vi "VI Server - 호출대상.vi"(7 "dB On (F)":bool caption="dB On (거짓)", 9 "export mode":T1 caption="반출 모드" items=["파워 스펙트럼", "파워 스펙트럼 밀도"], 10 "window":T2=1 caption="윈도우" items=["사각형"=0, "해닝"=1, "해밍"=2, "블랙맨-해리스"=3, "정밀한 블랙맨"=4, "블랙맨"=5, "플랫 탑(Flat Top)"=6, "4항 블랙맨-해리스 "=7, "7항 블랙맨-해리스"=8, "낮은 사이드로브"=9, "블랙맨 누탈"=11, "삼각파"=30, "바틀렛-해닝"=31, "보먼"=32, "파젠"=33, "웰치"=34, "카이저"=60, "돌프-체비셰프"=61, "가우스"=62], 11 "Frequency":dbl=10.1 caption="주파수") -> (1 "averages completed":dbl caption="완료된 평균", 3 "Power Spectrum / PSD":cluster{"f0":dbl, "df":dbl, "magnitude":dbl[]} caption="파워 스펙트럼 / PSD" {"magnitude" format="%.2p"; "f0" format="%0.2p"; "df" format="%0.2p"})   [LabVIEW 2014]
uses:
  <vilib>/Analysis/4window.llb/windowTd.ctl
  <vilib>/measure/maspectr.llb/Power Spectrum and PSD Export Mode.ctl
  <vilib>/measure/maspectr.llb/FFT Power Spectrum and PSD for 1 Chan.vi
  <vilib>/measure/NI_MAPro.lvlib
  <vilib>/Analysis/NI_AALPro.lvlib
panel:
  out "웨이브폼 그래프":cluster{"f0":dbl, "df":dbl, "magnitude":dbl[]}(graph)
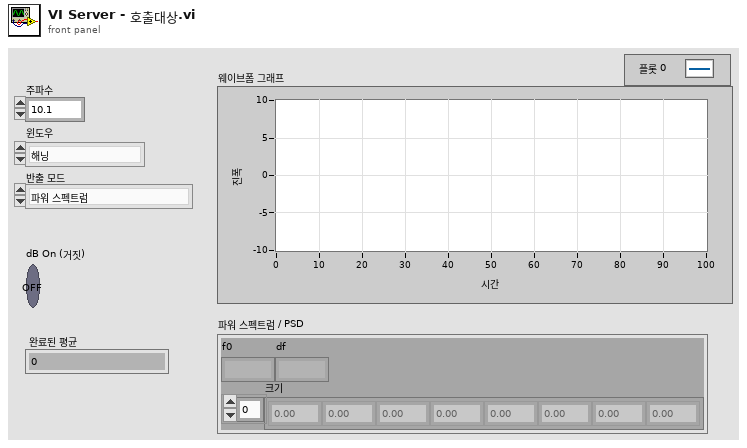
[diagram p1: front panel]
types:
  T1 = typedef "NI_MAPro.lvlib/Power Spectrum and PSD Export Mode.ctl" = u16
  T2 = typedef "NI_AALPro.lvlib/windowTd.ctl" = u32
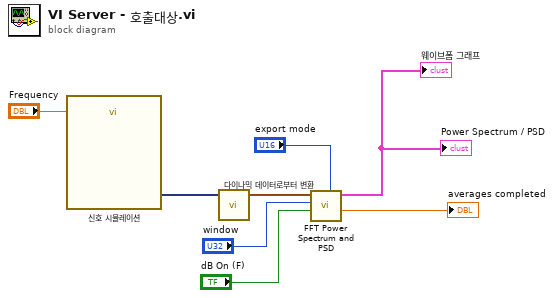
[diagram p0: block diagram]
diagram:
  n1 = call "신호 시뮬레이션"("Frequency"="Frequency") -> ("사인파"=w7:dynamicdata)  [unwired: 13 in, 1 out]
  n2 = call "다이나믹 데이터로부터 변환"("Dynamic Data Type"=w7) -> ("Waveform"=w6:waveform(dbl))  [unwired: 3 in]
  n3 = call-poly <vilib>:"FFT Power Spectrum and PSD.vi"("export mode"="export mode", "dB On (F)"="dB On (F)", "window"="window", "time signal"=w6) -> ("averages completed"=→"averages completed":dbl, "Power Spectrum / PSD"=→"Power Spectrum / PSD" →"웨이브폼 그래프":cluster{"f0":dbl, "df":dbl, "magnitude":dbl[]})  [unwired: 4 in, 2 out]
